vi "AFM_Driver_Manager.KillZombieProcesses.vi"(8 "error in (no error)":errorcluster, 11 "AFM_Driver_Manager in":refnum<class "AFM_Driver_Manager.lvclass">) -> (0 "error out":errorcluster, 3 "AFM_Driver_Manager out":refnum<class "AFM_Driver_Manager.lvclass">)   [LabVIEW 2019, in "AFM_Driver_Manager.lvclass"]
uses:
  AFM_Driver_Manager.lvclass
  AFM_Driver_Manager.lvclass/AFM_Driver_Manager.ctl
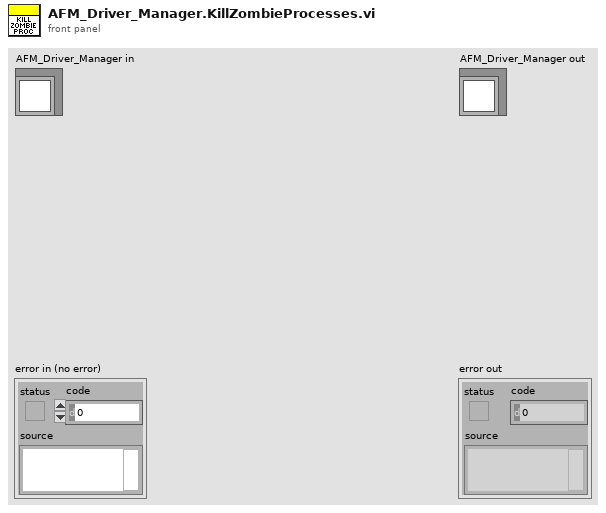
[diagram p1: front panel]
types:
  T1 = typedef "AFM_Driver_Manager.lvclass/AFM_Driver_Manager.PublicMethods.ctl" = cluster{"Stop Event":refnum<user-event>, "Lithography Data":refnum<user-event>, "Run Lithography":refnum<user-event>, "Background Image":refnum<user-event>, "Abort Notifier":refnum<user-event>}
  T2 = cluster{"VI Refnum":refnum<vi>, "Path":path, "Name":string, "Events":T1}[]
  T3 = enum32{"Bad", "Idle", "Run top level", "Running"}
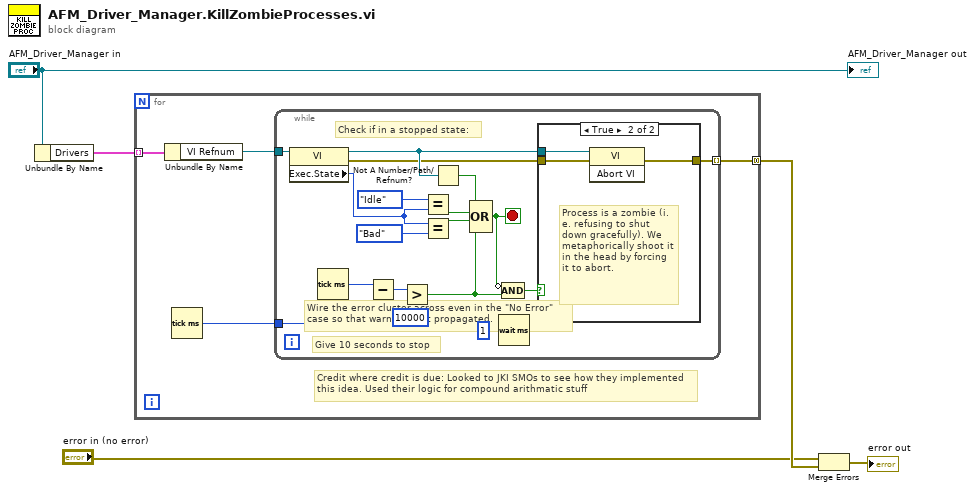
[diagram p0: block diagram]
diagram:
  # "Wire the error cluster across even in the \"No Error\"\ncase so that warnings get propagated."
  n1 = Unbundle By Name("AFM_Driver_Manager in") -> ("Drivers"=w5:T2)
  n2 = for {
    tunnel: w5 -> [w9] mode=indexing
    tunnel: [w6] -> w4 mode=concatenating
    # "Credit where credit is due: Looked to JKI SMOs to see how they implemented this idea. Used their logic for compound arithmatic stuff"
    n3 = Unbundle By Name(w9) -> ("VI Refnum"=w8:refnum<vi>)
    n4 = Tick Count (ms)() -> (millisecond timer value=w7:u32)
    n5 = while {
      tunnel: w7 -> [w19]
      tunnel: w8 -> [w27]
      tunnel: [w15] -> w6 mode=indexing
      stop <- w10 stop-if-true
      # "Check if in a stopped state:"
      # "Give 10 seconds to stop"
      n6 = property on="Property Node" class="VI"(reference=w27) -> (reference out=w17:refnum<vi>, error out=w12:errorcluster, "Exec.State"=w16:T3)  [unwired: 1 in]
      n7 = Tick Count (ms)() -> (millisecond timer value=w22:u32)
      n8 = Subtract(x=w22, y=w19) -> (x-y=w21:u32)
      n9 = Greater?(x=w21, y=u32 10000) -> (0:w13:bool)
      n10 = Equal?(x=T3."Idle", y=w16) -> (x = y?=w25:bool)
      n11 = Equal?(x=w16, y=T3."Bad") -> (x = y?=w23:bool)
      n12 = Not A Number/Path/Refnum?(number/path/refnum=w17) -> (NaN/Path/Refnum?=w14:bool)
      n13 = Compound Arithmetic op=OR(w14, w25, w23, w13) -> (w10:bool)
      n14 = Wait (ms)(milliseconds to wait=u32 1) -> ()  [unwired: 1 out]
      n15 = Compound Arithmetic op=AND(invert w10, w13) -> (w11:bool)
      n16 = case shown="True" w11 {
        tunnel: w17 -> [_ w31]
        tunnel: w12 -> [w28 w30]
        tunnel: [w28 w29] -> w15
        frame False {
          # "Timeout not reached yet."
        }
        frame True {
          # "Process is a zombie (i.e. refusing to shut down gracefully). We metaphorically shoot it in the head by forcing it to abort."
          n17 = invoke on="Invoke Node" class="VI" method="Abort VI"(reference=w31, error in=w30) -> (error out=w29:errorcluster)  [unwired: 1 in, 2 out]
        }
      }
    }
  }
  n18 = Merge Errors("error in (no error)", w4) -> (→"error out":errorcluster)
  "AFM_Driver_Manager out" <- "AFM_Driver_Manager in"
